vi "Simulacion_planta_control_PIDZiegler.vi"() -> ()   [LabVIEW 2012]
panel:
  out "sal_cont":dbl=61.25773808445103
  in  "c(k-3)":dbl
  in  "d4":dbl=-28.82
  in  "e(k-3)":dbl
  in  "c4":dbl=2.14
  in  "Entrada Deseada (RPM)":dbl=400.0
  in  "c(k-2)":dbl
  in  "c(k-1)":dbl
  in  "stop":bool
  in  "d1":dbl=28.82
  in  "d2":dbl=28.82
  in  "d3":dbl=-28.82
  in  "c1":dbl=2.482
  in  "c2":dbl=-2.128
  in  "c3":dbl=-2.47
  out "Entrada":dbl=0.006146024088081958
  in  "b1":dbl=1.0
  in  "b2":dbl=-1.96
  in  "b3":dbl=0.96
  in  "a1":dbl
  in  "a2":dbl=0.4164
  in  "a3":dbl=0.4168
  in  "Periodo":i32=10
  in  "e(k-2)":dbl
  in  "e(k-1)":dbl
  in  "Y(k-2)":dbl
  in  "Y(k-1)":dbl
  out "Salida y(k)":dbl(graph)=400.0061461228793
  # "MODELO DE LA PLANTA"
  # "Z  +"
  # "Z^2  +"
  # "Gp(z) = -------------------------------------------------------------------"
  # "Z^2  +"
  # "Z  +"
  # "CONTROLADOR"
  # "Z^2  +"
  # "Z  +"
  # "Z^3  +"
  # "Gp(z) = --------------------------------------------------------------------------------"
  # "Z ^2 +"
  # "Z  +"
  # "Z^3  +"
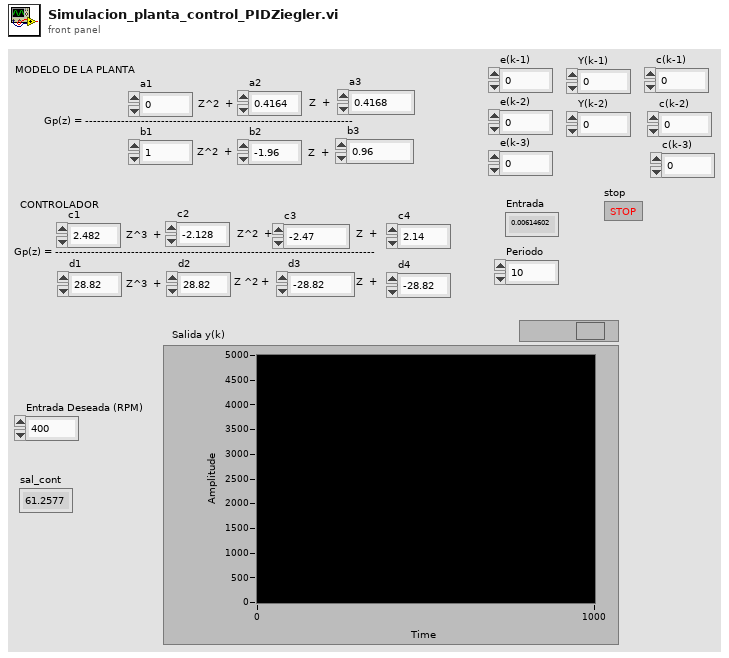
[diagram p1: front panel]
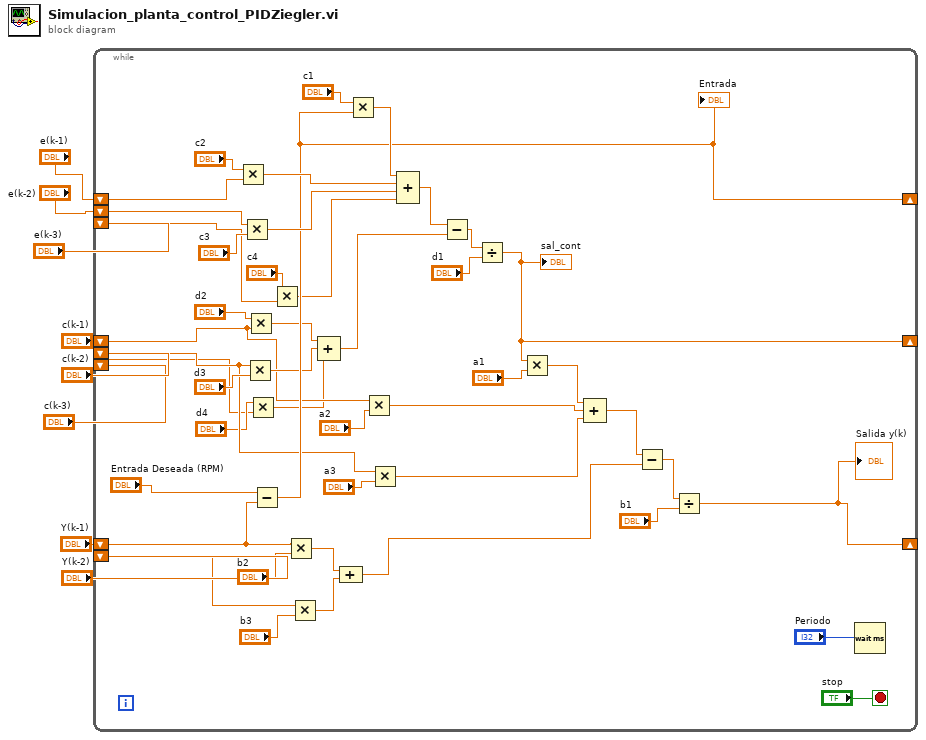
[diagram p0: block diagram]
diagram:
  n1 = while {
    shift-right: [w10] -> _
    shift-left: "Y(k-1)" -> [w40]
    shift-left: "Y(k-2)" -> [w49]
    shift-right: [w39] -> _
    shift-left: "e(k-1)" -> [w54]
    shift-left: "e(k-2)" -> [w53]
    shift-right: [w9] -> _
    shift-left: "c(k-1)" -> [w28]
    shift-left: "c(k-2)" -> [w26]
    shift-left: "e(k-3)" -> [w16]
    shift-left: "c(k-3)" -> [w13]
    stop <- "stop" stop-if-true
    n2 = Multiply(x="c2", y=w54) -> (x*y=w52:dbl)
    n3 = Multiply(x=w53, y="c3") -> (x*y=w51:dbl)
    n4 = Multiply(x=w26, y="d3") -> (x*y=w32:dbl)
    n5 = Multiply(x="d2", y=w28) -> (x*y=w33:dbl)
    n6 = Multiply(x="d4", y=w13) -> (x*y=w12:dbl)
    n7 = Subtract(x="Entrada Deseada (RPM)", y=w40) -> (x-y=w39:dbl)
    "Entrada" <- w39
    n8 = Multiply(x="c4", y=w16) -> (x*y=w15:dbl)
    n9 = Multiply(x=w40, y="b2") -> (x*y=w47:dbl)
    n10 = Multiply(x=w49, y="b3") -> (x*y=w46:dbl)
    n11 = Compound Arithmetic op=ADD(w33, w32, w12) -> (w31:dbl)
    n12 = Compound Arithmetic op=ADD(w47, w46) -> (w20:dbl)
    n13 = Multiply(x="c1", y=w39) -> (x*y=w43:dbl)
    n14 = Multiply(x=w28, y="a2") -> (x*y=w23:dbl)
    n15 = Multiply(x=w26, y="a3") -> (x*y=w22:dbl)
    n16 = Compound Arithmetic op=ADD(w43, w52, w51, w15) -> (w45:dbl)
    n17 = Subtract(x=w45, y=w31) -> (x-y=w44:dbl)
    n18 = Divide(x=w44, y="d1") -> (x/y=w9:dbl)
    "sal_cont" <- w9
    n19 = Multiply(x=w9, y="a1") -> (x*y=w24:dbl)
    n20 = Compound Arithmetic op=ADD(w24, w23, w22) -> (w21:dbl)
    n21 = Subtract(x=w21, y=w20) -> (x-y=w19:dbl)
    n22 = Divide(x=w19, y="b1") -> (x/y=w10:dbl)
    "Salida y(k)" <- w10
    n23 = Wait (ms)(milliseconds to wait="Periodo") -> ()  [unwired: 1 out]
  }
